vi "Scale Value (Exponent).vi"(11 "Value":dbl) -> (3 "Scaled Value":dbl)   [LabVIEW 2019, in "Audio Processing.lvlib"]
doc: "Scales the input value from range 0-1 to 0-20000, applying an exponential curve."
uses:
  Audio Processing.lvlib
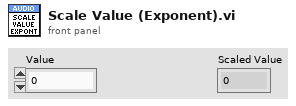
[diagram p1: front panel]
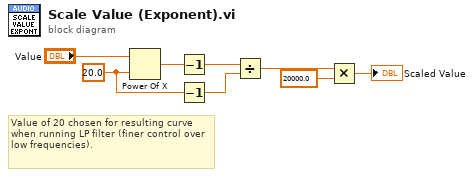
[diagram p0: block diagram]
diagram:
  w4 = 20.0 ("x")
  # "Value of 20 chosen for resulting curve when running LP filter (finer control over low frequencies)."
  n1 = Power Of X(1:w4, 2:"Value") -> (0:w5:dbl)
  n2 = Decrement(x=w5) -> (x-1=w8:dbl)
  n3 = Decrement(x=w4) -> (x-1=w3:dbl)
  n4 = Divide(x=w8, y=w3) -> (x/y=w7:dbl)
  n5 = Multiply(x=w7, y=20000.0) -> (x*y=→"Scaled Value":dbl)
